vi "nicrioDebugToken.vi"() -> ()   [LabVIEW 2020]
panel:
  out "text":string
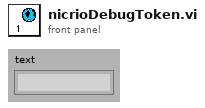
[diagram p1: front panel]
diagram:
